vi "Tx Core.vi"(0 "duc parameters":T1[](array[typedef]) {"frequency shift" format="%#.48g"}, 1 "tx.reset":bool=TRUE, 2 "fifo 0":refnum<k21>, 3 "fifo 1":refnum<k21>, 5 "tx.samples to generate":u32, 7 "tx.abort":bool, 9 "tx.stream enable":bool[](array[boolean]), 11 "tx.start trigger":bool) -> (4 "tx.state":T4, 6 "tx.samples processed":u32, 8 "tx.number of fifo underflows":u32, 10 "tx.number of iq data overflows":u64[](array[numeric]), 14 "tx.dsp reset done":bool)   [LabVIEW 2020]
uses:
  Stream Control State.ctl
  DUC Parameters.ctl
  <instrlib>/_niInstr/DSP/v1/Shared/Public/IQ Impairments.ctl
  <instrlib>/_niInstr/DSP/v1/Shared/Public/IQ Gain.ctl
  <vilib>/rvi/eio/common/nirviEmuTemplateMethod_errors.vi
  <vilib>/eio/EIONode/EIONode.xnode
  <instrlib>/_niInstr/Basic Elements/v1/FPGA/niInstr Basic Elements v1 FPGA.lvlib
  <instrlib>/_niInstr/DSP/v1/Shared/niInstr DSP v1 Shared.lvlib
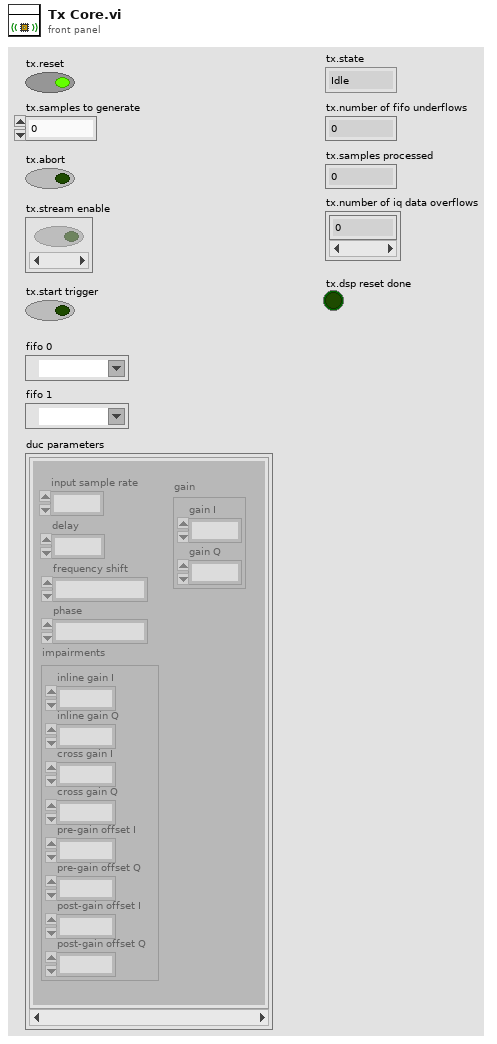
[diagram p1: front panel]
types:
  T1 = typedef "DUC Parameters.ctl" = cluster{"frequency shift":fxp<+/-,48,0>, "impairments":T2, "phase":fxp<+/-,21,0>, "input sample rate":fxp<+,48,1>, "gain":T3, "delay":fxp<+/-,18,0>}
  T2 = typedef "niInstr DSP v1 Shared.lvlib/IQ Impairments.ctl" = cluster{"inline gain I":fxp<+/-,18,1>, "inline gain Q":fxp<+/-,18,1>, "cross gain I":fxp<+/-,18,1>, "cross gain Q":fxp<+/-,18,1>, "pre-gain offset I":fxp<+/-,18,1>, "pre-gain offset Q":fxp<+/-,18,1>, "post-gain offset I":fxp<+/-,18,1>, "post-gain offset Q":fxp<+/-,18,1>}
  T3 = typedef "niInstr DSP v1 Shared.lvlib/IQ Gain.ctl" = cluster{"gain I":fxp<+/-,24,3>, "gain Q":fxp<+/-,24,3>}
  T4 = typedef "Stream Control State.ctl" = enum16{"Idle", "Active"}
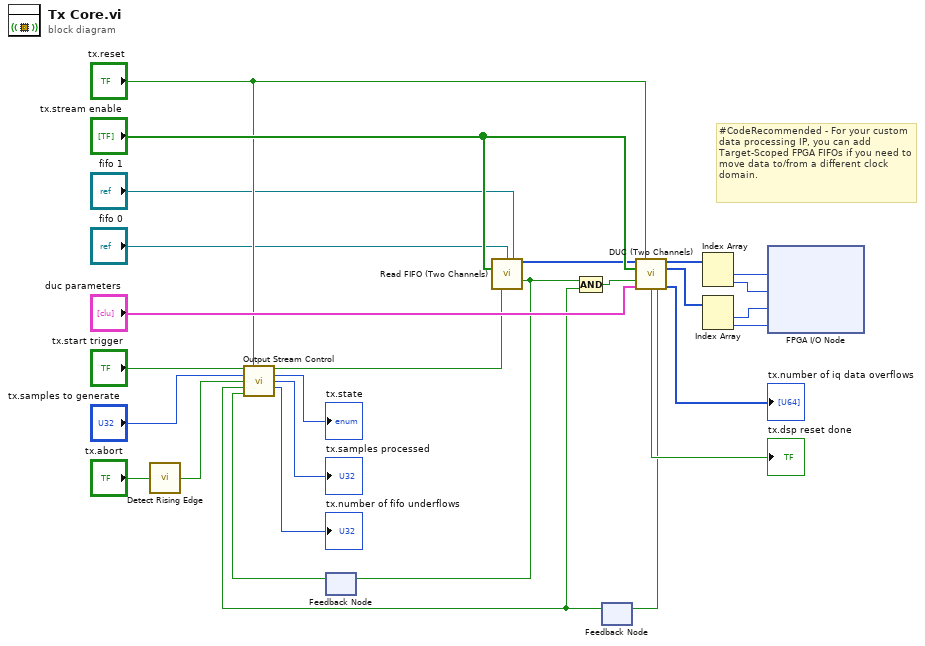
[diagram p0: block diagram]
diagram:
  # "#CodeRecommended - For your custom data processing IP, you can add Target-Scoped FPGA FIFOs if you need to move data to/from a different clock domain."
  n1 = call <instrlib>:"Detect Rising Edge.vi"("signal"="tx.abort") -> ("edge detected"=w14:bool)  [unwired: 14 in]
  n2 = feedback #1() -> (w10:bool)  [unwired: 1 in]
  n3 = feedback #2() -> (w12:bool)  [unwired: 1 in]
  n4 = call "Output Stream Control.vi"("start trigger"="tx.start trigger", "reset"="tx.reset", "burst size"="tx.samples to generate", "abort"=w14, "ready to read stream (T)"=w12, "fifo output valid"=w10) -> ("read stream"=w2:bool, "state"=→"tx.state":T4, "samples processed"=→"tx.samples processed":u32, "number of underflows"=→"tx.number of fifo underflows":u32)  [unwired: 5 in, 1 out]
  n5 = call "Read FIFO (Two Channels).vi"("fifo 0"="fifo 0", "fifo 1"="fifo 1", "enable"="tx.stream enable", "ready for output"=w2) -> ("data"=w4:u32[], "output valid"=w3:bool)  [unwired: 10 in]
  n6 = feedback-in #1(w3) -> ()
  n7 = Compound Arithmetic op=AND(w3, w12) -> (w25:bool)
  n8 = call "DUC (Two Channels).vi"("data"=w4, "reset"="tx.reset", "enable"="tx.stream enable", "input valid"=w25, "duc parameters"="duc parameters") -> ("I data out"=w17:i16[], "Q data out"=w19:i16[], "dsp reset done"=→"tx.dsp reset done":bool, "ready for input"=w15:bool, "number of overflows"=→"tx.number of iq data overflows":u64[])  [unwired: 6 in]
  n9 = feedback-in #2(w15) -> ()
  n10 = Index Array(array=w17) -> (element #1=w18:i16, element #2=w21:i16)  [unwired: 2 in]
  n11 = Index Array(array=w19) -> (element #1=w22:i16, element #2=w23:i16)  [unwired: 2 in]
  n12 = xnode "FPGA I/O Node"("RF 0/Tx/I"=w18, "RF 1/Tx/I"=w21, "RF 0/Tx/Q"=w22, "RF 1/Tx/Q"=w23) -> ()  [unwired: 4 in, 4 out]
